vi "Write Config.vi"(8 "error in (no error)":errorcluster, 9 "Re-Init?":bool, 10 "ICM File In":path, 11 "NI DA in":refnum<class "NI Digital to Analog.lvclass">) -> (0 "error out":errorcluster, 3 "NI DA out":refnum<class "NI Digital to Analog.lvclass">)   [LabVIEW 2018, in "NI Digital to Analog.lvclass"]
doc: "NI Analog.lvclass:Write Config.vi\n\nThis VI writes the NI Analog Class parameters to the ICM configuration file.\n\nInstrument Communication Module Version 1.0\nJanuary, 2018 Original Code Consulting David Thomson\n www.originalcode.com"
uses:
  NI Digital to Analog.lvclass
  NI Digital to Analog.lvclass/NI Digital to Analog.ctl
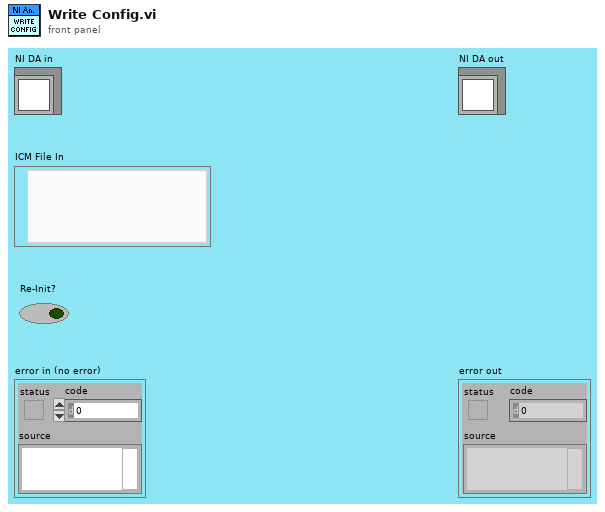
[diagram p1: front panel]
types:
  T1 = typedef "NI Analog Config.ctl" = cluster{"Device":string, "SE/Diff":bool, "Channels":cluster{"Channel":i32, "Range":T2}[]}
  T2 = typedef "NI Analog Channel Range.ctl" = enum16{"-10.0 to 10.0 V", "-5.0 to 5.0 V", "-2.0 to 2.0 V", "-1.0 to 1.0 V", "-0.5 to 0.5 V", "-0.2 to 0.2 V", "-0.1 to 0.1 V", "0 to 10 V", "0 to 5 V", "0 to 2 V", "0 to 1 V", "0 to 0.5 V", "0 to 0.2 V", "0 to 0.1 V"}
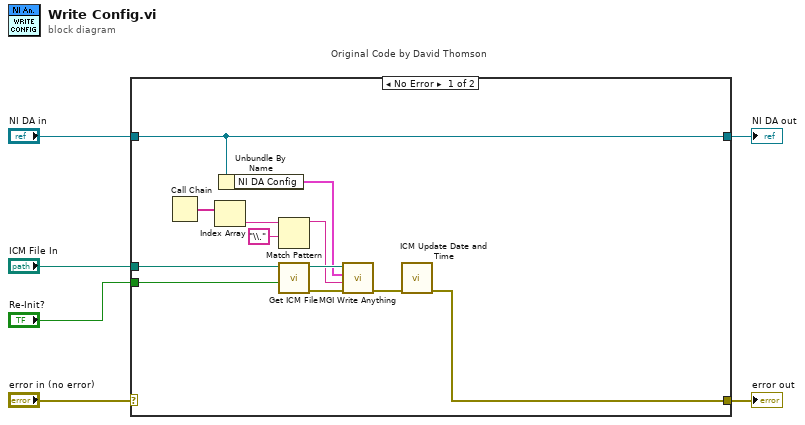
[diagram p0: block diagram]
diagram:
  n1 = case "Original Code by David Thomson" shown="No Error" "error in (no error)" {
    selector: "error in (no error)" -> [_ w20]
    tunnel: [w7 w20] -> w5
    tunnel: [w15 w19] -> w3
    tunnel: "NI DA in" -> [w15 w19]
    tunnel: "ICM File In" -> [w10 _]
    tunnel: "Re-Init?" -> [w9 _]
    frame No Error {
      n2 = Call Chain() -> (call chain=w17:string[])
      n3 = Index Array(array=w17) -> (element=w16:string)  [unwired: 1 in]
      n4 = Unbundle By Name(w15) -> ("NI DA Config"=w11:T1)
      n5 = Match Pattern(string=w16, regular expression="\\.") -> (before substring=w12:string)  [unwired: 1 in, 3 out]
      n6 = call "Get ICM File.vi"("Re-Init?"=w9, "ICM File In"=w10) -> ("error out"=w14:errorcluster, "ICM File"=w13:path)  [unwired: 8 in]
      n7 = call "MGI Write Anything.vi"("Error In"=w14, "Section Name (Name of \"Anything\")"=w12, "Anything"=w11, "Path (dialog)"=w13) -> ("Error Out"=w8:errorcluster)  [unwired: 5 in, 2 out]
      n8 = call "ICM Update Date and Time.vi"("error in (no error)"=w8) -> ("error out"=w7:errorcluster)  [unwired: 9 in, 1 out]
    }
    frame Error {
    }
  }
  "error out" <- w5
  "NI DA out" <- w3
